vi "FTW-Actor-Initialize.vi"(0 "FTW Actor Instance Type":refnum<class "FTW-ActorInstance.lvclass">, 5 "Initialization Job Sequence":string, 7 "Actor Instance Configuration":T1, 11 "error in":errorcluster) -> (4 "FTW Actor Instance":refnum<class "FTW-ActorInstance.lvclass">, 6 "Incoming Requests":refnum<event-registration>, 15 "error out":errorcluster)   [LabVIEW 2012, in "FTW-Actor.lvlib" / "FTW-ActorInstance.lvclass"]
uses:
  FTW-ActorInstance.lvclass
  Utility/FTW-Actor-Configuration.ctl
  Message/Request/FTW-Message-IncomingRequest.lvclass
  Utility/FTW-Actor-Address.ctl
  FTW-ActorInstance.lvclass/FTW-ActorInstance.ctl
  Endpoint/FTW-Endpoint.lvclass
  Core/src/Reflection/FTW-Reflection-Type.vi
  Core/src/JSON/FTW-JSON-Core-LibraryFilepath.vi
  Core/src/JSON/FTW-JSON-Core-GetFlattenedValue.vi
  Core/src/JSON/FTW-JSON-Core-LibraryError.vi
  Core/utils/CodeGen/JSON Deserialize/FTW-JSON-Deserialize.xnode
  JobSequencer/FTW-JobSequencer.lvclass
  Ether/FTW-Ether.lvclass
  FTW-Actor.lvlib
  EventLogger/FTW-Logger.lvclass
panel:
  # "Inputs"
  # "Outputs"
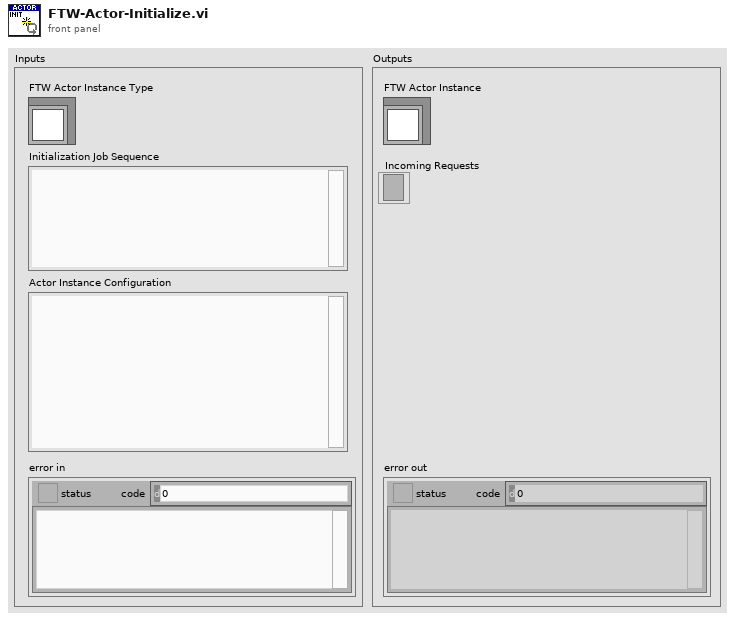
[diagram p1: front panel]
types:
  T1 = typedef "FTW-Actor.lvlib/FTW-Actor-Configuration.ctl" = string
  T2 = typedef "FTW-Actor.lvlib/FTW-Actor-Address.ctl" = string
  T3 = cluster{"Identity":string, "DebugEnableInboxLogging":bool, "DebugEnableJobLogging":bool, "InboxAddress":T2, "PublisherAddress":T2, "LoggerAddress":T2, "LauncherAddress":T2}
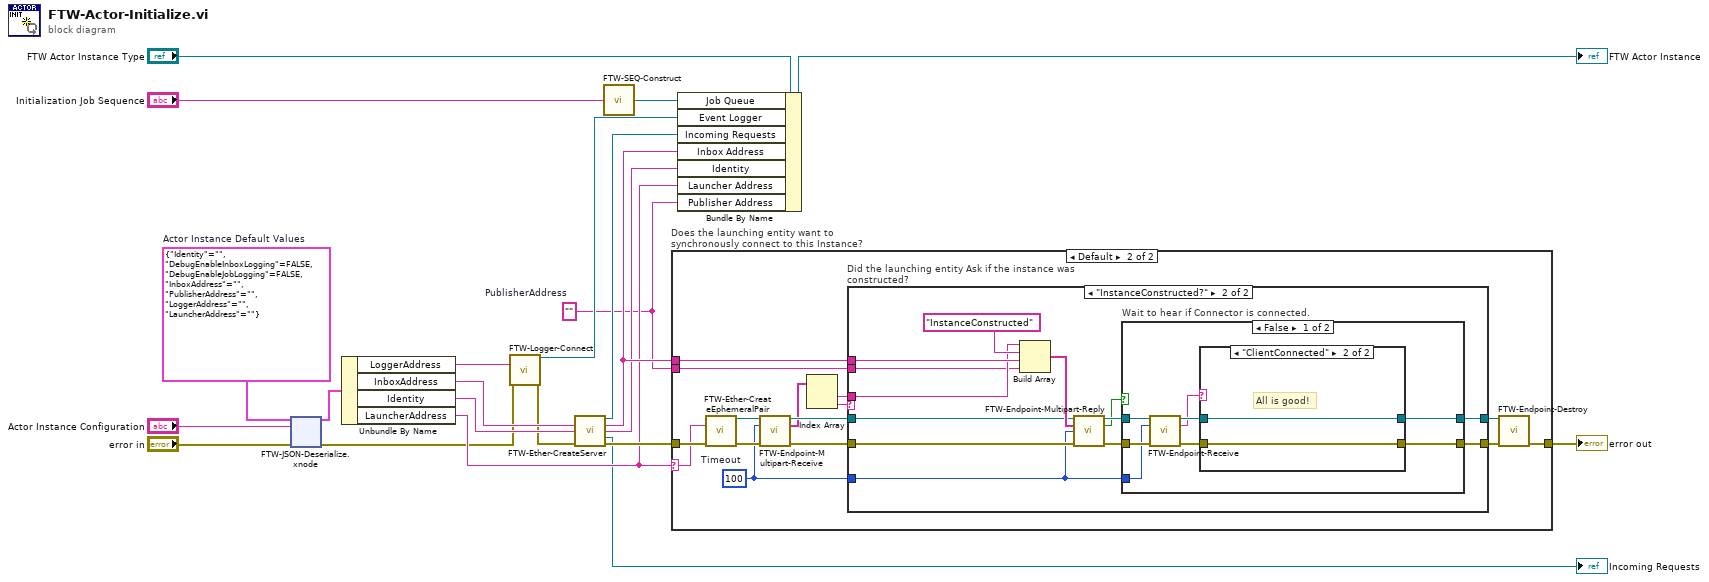
[diagram p0: block diagram]
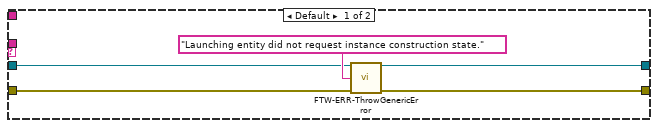
[diagram p3: hidden frame]
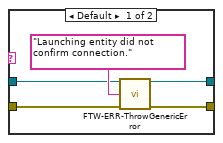
[diagram p4: hidden frame]
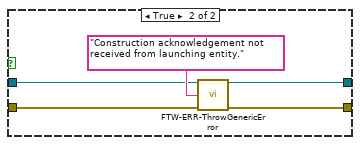
[diagram p5: hidden frame]
diagram:
  w11 = T2 ""  # PublisherAddress
  w2 = T3 {"Identity"="", "DebugEnableInboxLogging"=FALSE, "DebugEnableJobLogging"=FALSE, "InboxAddress"="", "PublisherAddress"="", "LoggerAddress"="", "LauncherAddress"=""}  # Actor Instance Default Values
  n1 = xnode "FTW-JSON-Deserialize.xnode"("Type and Defaults"=w2, "JSON String"="Actor Instance Configuration", "error in"="error in") -> ("Values"=w1:T3, "error out"=w3:errorcluster)
  n2 = Unbundle By Name(w1) -> ("LoggerAddress"=w14:T2, "InboxAddress"=w18:T2, "Identity"=w17:string, "LauncherAddress"=w12:T2)
  n3 = call "FTW-Logger-Connect.vi"("Logger Address"=w14, "error in"=w3) -> ("FTW Logger Connector"=w16:refnum<class "FTW-Logger.lvclass">, "error out"=w15:errorcluster)  [unwired: 12 in]
  n4 = call "FTW-Ether-CreateServer.vi"("Server Address"=w18, "Server Identity"=w17, "error in"=w15) -> ("Server Endpoint"=w20:refnum<class "FTW-Endpoint.lvclass">, "Actual Server Address"=w22:T2, "Actual Identity"=w19:string, "Incoming Requests"=→"Incoming Requests":refnum<event-registration>, "error out"=w13:errorcluster)  [unwired: 8 in]
  n5 = call "FTW-SEQ-Construct.vi"("Initial Sequence"="Initialization Job Sequence") -> ("FTW Job Sequencer"=w21:refnum<class "FTW-JobSequencer.lvclass">)
  n6 = case "Does the launching entity want to synchronously connect to this Instance?" shown="Default" w12 {
    selector: w12 -> [_ w25]
    tunnel: w13 -> [w23 w28]
    tunnel: w22 -> [_ w38]
    tunnel: [w23 w31] -> w9
    tunnel: w11 -> [_ w26]
    frame "" {
    }
    frame Default {
      w24 = 100  # Timeout
      n7 = call "FTW-Ether-CreateEphemeralPair.vi"("Requested Ephemeral Address"=w25, "error in"=w28) -> ("Ephemeral Endpoint"=w29:refnum<class "FTW-Endpoint.lvclass">, "error out"=w27:errorcluster)  [unwired: 11 in, 1 out]
      n8 = call-dynamic "FTW-Endpoint-Multipart-Receive.vi"("FTW Endpoint"=w29, "Timeout"=w24, "error in"=w27) -> ("FTW Endpoint out"=w36:refnum<class "FTW-Endpoint.lvclass">, "Message Received"=w35:string[], "error out"=w37:errorcluster)  [unwired: 9 in, 1 out]
      n9 = Index Array(array=w35) -> (element #1=w33:string, element #2=w34:string)  [unwired: 2 in]
      n10 = case "Did the launching entity Ask if the instance was constructed?" shown="\"InstanceConstructed?\"" w34 {
        tunnel: w38 -> [_ w55]
        tunnel: w37 -> [w42 w52]
        tunnel: w36 -> [w39 w51]
        tunnel: w33 -> [_ w50]
        tunnel: [w41 w47] -> w30
        tunnel: [w39 w45] -> w32
        tunnel: w26 -> [_ w44]
        tunnel: w24 -> [_ w43]
        frame Default {
          n11 = call "FTW-ERR-ThrowGenericError.vi"("Error Message"="Launching entity did not request instance construction state.", "error in"=w42) -> ("error out"=w41:errorcluster)  [unwired: 13 in]
        }
        frame "InstanceConstructed?" {
          n12 = Build Array(w50, "InstanceConstructed", w55, w44) -> (w53:T2[])
          n13 = call-dynamic "FTW-Endpoint-Multipart-Reply.vi"("FTW Endpoint"=w51, "Multipart Message"=w53, "Timeout"=w43, "error in"=w52) -> ("FTW Endpoint out"=w49:refnum<class "FTW-Endpoint.lvclass">, "Timed out?"=w46:bool, "error out"=w48:errorcluster)  [unwired: 9 in]
          n14 = case "Wait to hear if Connector is connected." shown="False" w46 {
            tunnel: w49 -> [w61 w70]
            tunnel: w48 -> [w59 w72]
            tunnel: w43 -> [w58 _]
            tunnel: [w62 w71] -> w47
            tunnel: [w63 w70] -> w45
            frame False {
              n15 = call-dynamic "FTW-Endpoint-Receive.vi"("FTW Endpoint"=w61, "Timeout"=w58, "error in"=w59) -> ("FTW Endpoint out"=w60:refnum<class "FTW-Endpoint.lvclass">, "Message Header"=w56:string, "error out"=w57:errorcluster)  [unwired: 8 in, 2 out]
              n16 = case shown="\"ClientConnected\"" w56 {
                tunnel: w60 -> [w65 w69]
                tunnel: w57 -> [w66 w68]
                tunnel: [w65 w69] -> w63
                tunnel: [w64 w68] -> w62
                frame Default {
                  n17 = call "FTW-ERR-ThrowGenericError.vi"("Error Message"="Launching entity did not confirm connection.", "error in"=w66) -> ("error out"=w64:errorcluster)  [unwired: 13 in]
                }
                frame "ClientConnected" {
                  # "All is good!"
                }
              }
            }
            frame True {
              n18 = call "FTW-ERR-ThrowGenericError.vi"("Error Message"="Construction acknowledgement not received from launching entity.", "error in"=w72) -> ("error out"=w71:errorcluster)  [unwired: 13 in]
            }
          }
        }
      }
      n19 = call-dynamic "FTW-Endpoint-Destroy.vi"("FTW Endpoint"=w32, "error in"=w30) -> ("error out"=w31:errorcluster)  [unwired: 13 in]
    }
  }
  "error out" <- w9
  n20 = Bundle By Name(cluster="FTW Actor Instance Type", "Job Queue"=w21, "Event Logger"=w16, "Incoming Requests"=w20, "Inbox Address"=w22, "Identity"=w19, "Launcher Address"=w12, "Publisher Address"=w11) -> (→"FTW Actor Instance":refnum<class "FTW-ActorInstance.lvclass">)
